vi "Queue Driver.vi"(0 "Enqueue":T1, 1 "Queue Name":string, 5 "Enqueue-N":T1[](array[typedef]), 11 "error in":errorcluster, 13 "Queue Operations":T2) -> (4 "Dequued Element":T1, 15 "error out":errorcluster)   [LabVIEW 2020]
doc: "This VI is used to perform Queue operations. Basically it acts as a Queue driver."
uses:
  Typedefs/Queue Operations.ctl
  Typedefs/Queue State.ctl
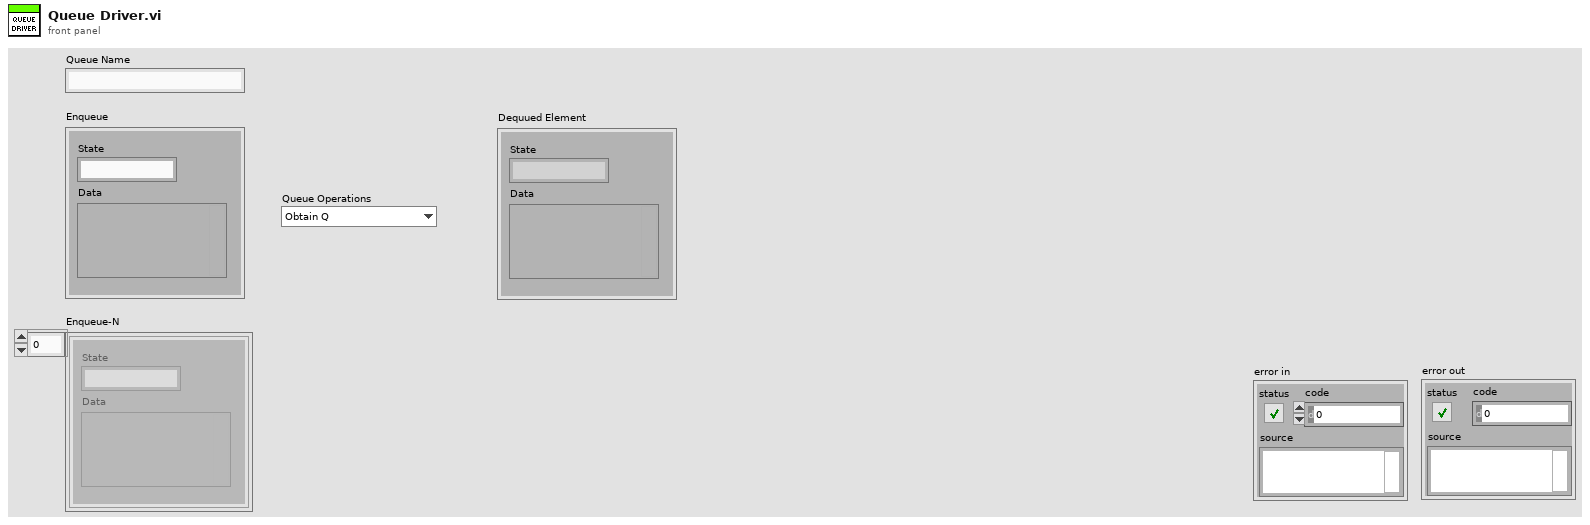
[diagram p1: front panel]
types:
  T1 = typedef "Queue State.ctl" = cluster{"State":string, "Data":variant}
  T2 = typedef "Queue Operations.ctl" = enum16{"Obtain Q", "EnQ", "EnQ-N", "DeQ", "EnStack", "Flush-Q", "Release Q"}
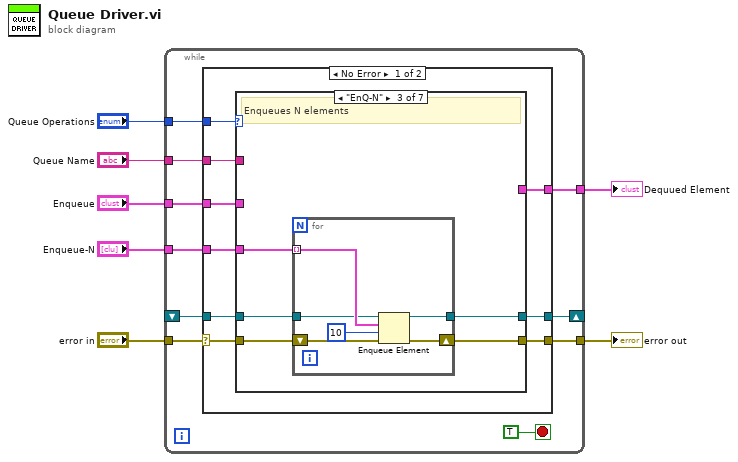
[diagram p0: block diagram]
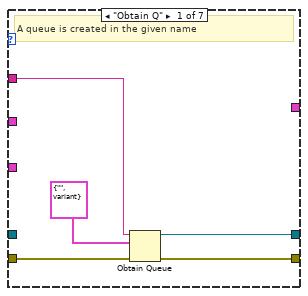
[diagram p2: hidden frame]
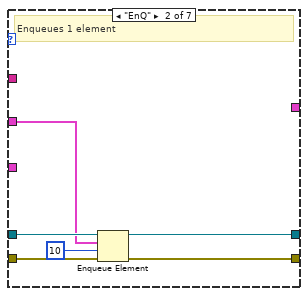
[diagram p3: hidden frame]
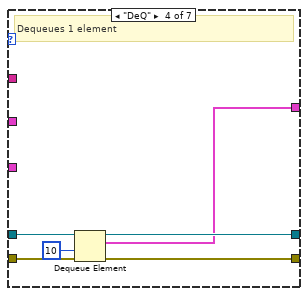
[diagram p4: hidden frame]
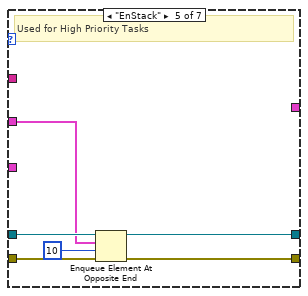
[diagram p5: hidden frame]
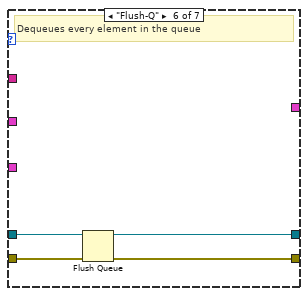
[diagram p6: hidden frame]
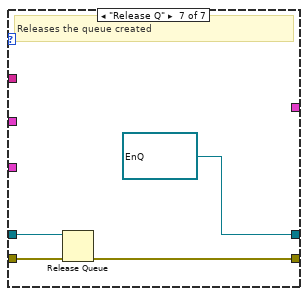
[diagram p7: hidden frame]
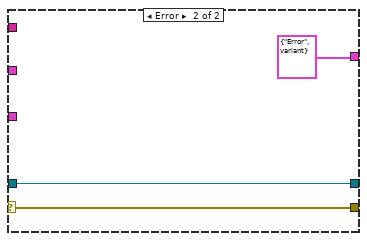
[diagram p8: hidden frame]
diagram:
  n1 = while {
    tunnel: "Queue Operations" -> [w17]
    tunnel: "error in" -> [w16]
    tunnel: [w15] -> w5
    shift-right: [w12] -> _
    shift-left: _ -> [w11]
    tunnel: "Queue Name" -> [w13]
    tunnel: "Enqueue" -> [w10]
    tunnel: "Enqueue-N" -> [w9]
    tunnel: [w8] -> w1
    stop <- TRUE stop-if-true
    n2 = case shown="No Error" w16 {
      selector: w16 -> [w25 w71]
      tunnel: w17 -> [w26 _]
      tunnel: [w24 w71] -> w15
      tunnel: w13 -> [w23 _]
      tunnel: [w22 w70] -> w12
      tunnel: w11 -> [w21 w70]
      tunnel: w10 -> [w20 _]
      tunnel: w9 -> [w19 _]
      tunnel: [w18 cluster{"State":string, "Data":variant} {"State"="Error", "Data"=variant} ("EnQ")] -> w8
      frame No Error {
        n3 = case shown="\"EnQ-N\"" w26 {
          tunnel: w25 -> [w31 w37 w42 w54 w60 w64 w68]
          tunnel: [w30 w36 w41 w53 w59 w63 w67] -> w24
          tunnel: w23 -> [w28 _ _ _ _ _ _]
          tunnel: [w27 w33 w38 w50 w57 w61 refnum<queue> refnum ("queue out")] -> w22
          tunnel: w21 -> [_ w34 w39 w51 w56 w62 w66]
          tunnel: w20 -> [_ w32 _ _ w55 _ _]
          tunnel: w19 -> [_ _ w40 _ _ _ _]
          tunnel: [_ _ _ w49 _ _ _] -> w18
          frame "Obtain Q" {
            # "A queue is created in the given name"
            n4 = Obtain Queue(name (unnamed)=w28, element data type=T1 {"State"="", "Data"=variant} ("EnQ"), error in (no error)=w31) -> (queue out=w27:refnum<queue>, error out=w30:errorcluster)  [unwired: 2 in, 1 out]
          }
          frame "EnQ" {
            # "Enqueues 1 element"
            n5 = Enqueue Element(queue=w34, element=w32, timeout in ms (-1)=10, error in (no error)=w37) -> (queue out=w33:refnum<queue>, error out=w36:errorcluster)  [unwired: 1 out]
          }
          frame "EnQ-N" {
            # "Enqueues N elements"
            n6 = for {
              shift-right: [w47] -> w41
              shift-left: w42 -> [w48]
              tunnel: [w45] -> w38
              tunnel: w40 -> [w44] mode=indexing
              tunnel: w39 -> [w43]
              n7 = Enqueue Element(queue=w43, element=w44, timeout in ms (-1)=10, error in (no error)=w48) -> (queue out=w45:refnum<queue>, error out=w47:errorcluster)  [unwired: 1 out]
            }
          }
          frame "DeQ" {
            # "Dequeues 1 element"
            n8 = Dequeue Element(queue=w51, timeout in ms (-1)=10, error in (no error)=w54) -> (queue out=w50:refnum<queue>, element=w49:T1, error out=w53:errorcluster)  [unwired: 1 out]
          }
          frame "EnStack" {
            # "Used for High Priority Tasks"
            n9 = Enqueue Element At Opposite End(queue=w56, element=w55, timeout in ms (-1)=10, error in (no error)=w60) -> (queue out=w57:refnum<queue>, error out=w59:errorcluster)  [unwired: 1 out]
          }
          frame "Flush-Q" {
            # "Dequeues every element in the queue"
            n10 = Flush Queue(queue=w62, error in (no error)=w64) -> (queue out=w61:refnum<queue>, error out=w63:errorcluster)  [unwired: 1 out]
          }
          frame "Release Q" {
            # "Releases the queue created"
            n11 = Release Queue(queue=w66, error in (no error)=w68) -> (error out=w67:errorcluster)  [unwired: 1 in, 2 out]
          }
        }
      }
      frame Error {
      }
    }
  }
  "error out" <- w5
  "Dequued Element" <- w1
